vi "Get Number of Click Zones.vi"(11 "array in":T2) -> (2 "number of click zones":i32, 3 "array out":T2)   [LabVIEW 2017, in "NI_Robotics_Configure Steering Frame.lvlib"]
uses:
  <vilib>/robotics/Dialog/Configure Steering Frame/NI_Robotics_Configure Steering Frame.lvlib
  <vilib>/robotics/Dialog/Configure Steering Frame/Click Zone.ctl
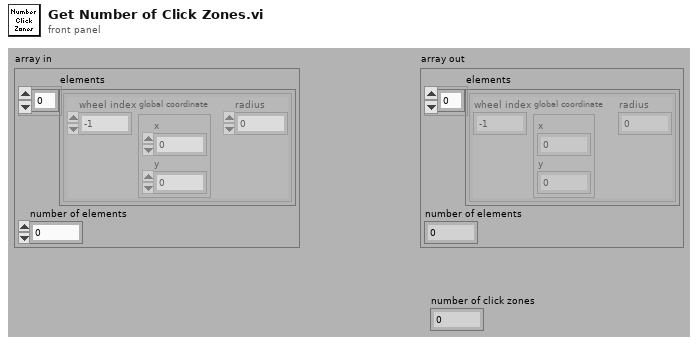
[diagram p1: front panel]
types:
  T1 = typedef "NI_Robotics_Configure Steering Frame.lvlib/Click Zone.ctl" = cluster{"wheel index":i32, "global coordinate":cluster{"x":dbl, "y":dbl}, "radius":dbl}
  T2 = cluster{"elements":T1[], "number of elements":i32}
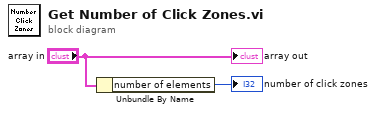
[diagram p0: block diagram]
diagram:
  n1 = Unbundle By Name("array in") -> ("number of elements"=→"number of click zones":i32)
  "array out" <- "array in"
